vi "Set Line Filter.vi"(8 "error in (no error)":errorcluster, 10 "Line Frequency Rejection":T1, 11 "VISA resource name":refnum<visa-resource-name>) -> (0 "error out":errorcluster, 3 "VISA resource name out":refnum<visa-resource-name>)   [LabVIEW 2016, in "SR7270 Drivers.lvclass"]
uses:
  SR7270 Drivers.lvclass
  Typedefs/LF--enum.ctl
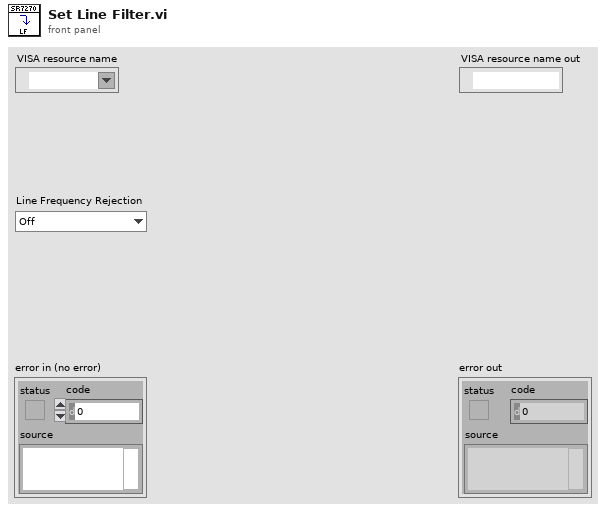
[diagram p1: front panel]
types:
  T1 = typedef "SR7270 Drivers.lvclass/LF--enum.ctl" = enum16{"Off", "60 Hz", "120 Hz", "60 & 120 Hz"}
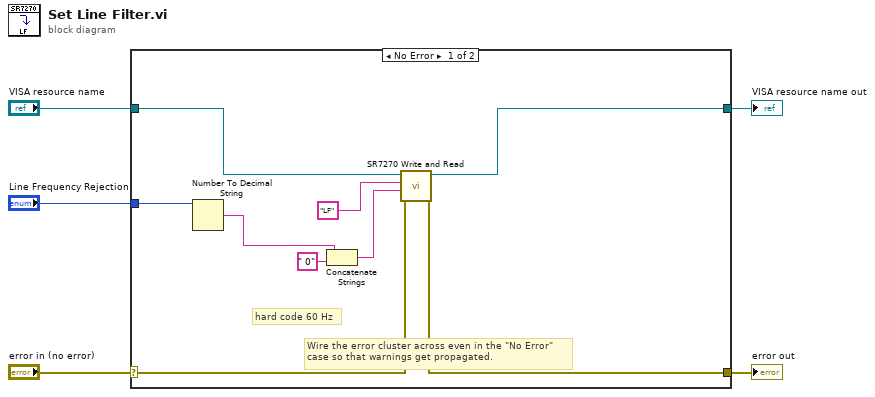
[diagram p0: block diagram]
diagram:
  n1 = case shown="No Error" "error in (no error)" {
    selector: "error in (no error)" -> [w14 w16]
    tunnel: [w13 w16] -> w4
    tunnel: [w6 w15] -> w2
    tunnel: "VISA resource name" -> [w7 w15]
    tunnel: "Line Frequency Rejection" -> [w11 _]
    frame No Error {
      # "hard code 60 Hz"
      # "Wire the error cluster across even in the \"No Error\"\ncase so that warnings get propagated."
      n2 = Number To Decimal String(number=w11) -> (decimal integer string=w9:string)  [unwired: 1 in]
      n3 = Concatenate Strings(w9, " 0" ("string")) -> (w8:string)
      n4 = call "SR7270 Write and Read.vi"("error in (no error)"=w14, "Parameter(s)"=w8, "Command Name"="LF", "VISA resource name"=w7) -> ("error out"=w13:errorcluster, "VISA resource name out"=w6:refnum<visa-resource-name>)  [unwired: 4 in, 2 out]
    }
    frame Error {
    }
  }
  "error out" <- w4
  "VISA resource name out" <- w2
